vi "Graph Value.vi"(2 "Minimum?":bool, 3 "Input":dbl) -> (0 "Min/max":dbl, 1 "Output":dbl)   [LabVIEW 2013]
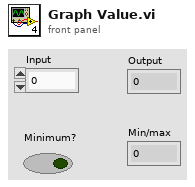
[diagram p1: front panel]
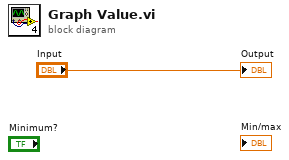
[diagram p0: block diagram]
diagram:
  "Output" <- "Input"
